vi "GetSwerveEncoders.vi"() -> (16 "Swerve 0 Velocity (ft/s)":dbl, 17 "Swerve 3 Velocity (ft/s)":dbl, 18 "Swerve 1 Velocity (ft/s)":dbl, 19 "Swerve 2 Velocity (ft/s)":dbl, 20 "Swerve 0 Azimuth Position (deg)":dbl, 22 "Swerve 1 Azimuth Position (deg)":dbl, 24 "Swerve 2 Azimuth Position (deg)":dbl, 26 "Swerve 3 Azimuth Position (deg)":dbl)   [LabVIEW 2020]
doc: "Gets the drive distance, azimuth position, and velocity encoder readings from all of the swerve modules. This VI is also useful for characterizing the drive system allowing for estimation of the robot acceleration and plotting of the module velocities. Deteremines the true shifter state based on photo-interrupter sensors on each module. Please see sensors.vi for a reading of the true robot ground speed (as this must be calculated after using the module odometry VIs)."
uses:
  driverdata.vi
  refnums.vi
  GRNF_CTREMotor.vi
  <vilib>/Rock Robotics/WPI/ThirdParty/Phoenix-LabVIEW/Motor Controller/Get/CTRE_Phoenix_MotorController_GetGeneralStatus.vi
  <vilib>/Rock Robotics/WPI/ThirdParty/Phoenix-LabVIEW/Motor Controller/Get/CTRE_Phoenix_MotorController_GetLimitSwitchStates.vi
  <vilib>/Rock Robotics/WPI/ThirdParty/Phoenix-LabVIEW/Motor Controller/Get/CTRE_Phoenix_MotorController_GetSelectedSensorData.vi
  sensors.vi
panel:
  in  "Shift Time Threshold (ms)":u32=250
  out "Acceleration (ft/s^2)":dbl format="%.1f"
  in  "Reset Acceleration Test":bool
  in  "Plot and Measure":bool
  out "Drive Encoder Velocities (ft/s)":cluster{dbl, dbl, dbl, dbl}(graph)
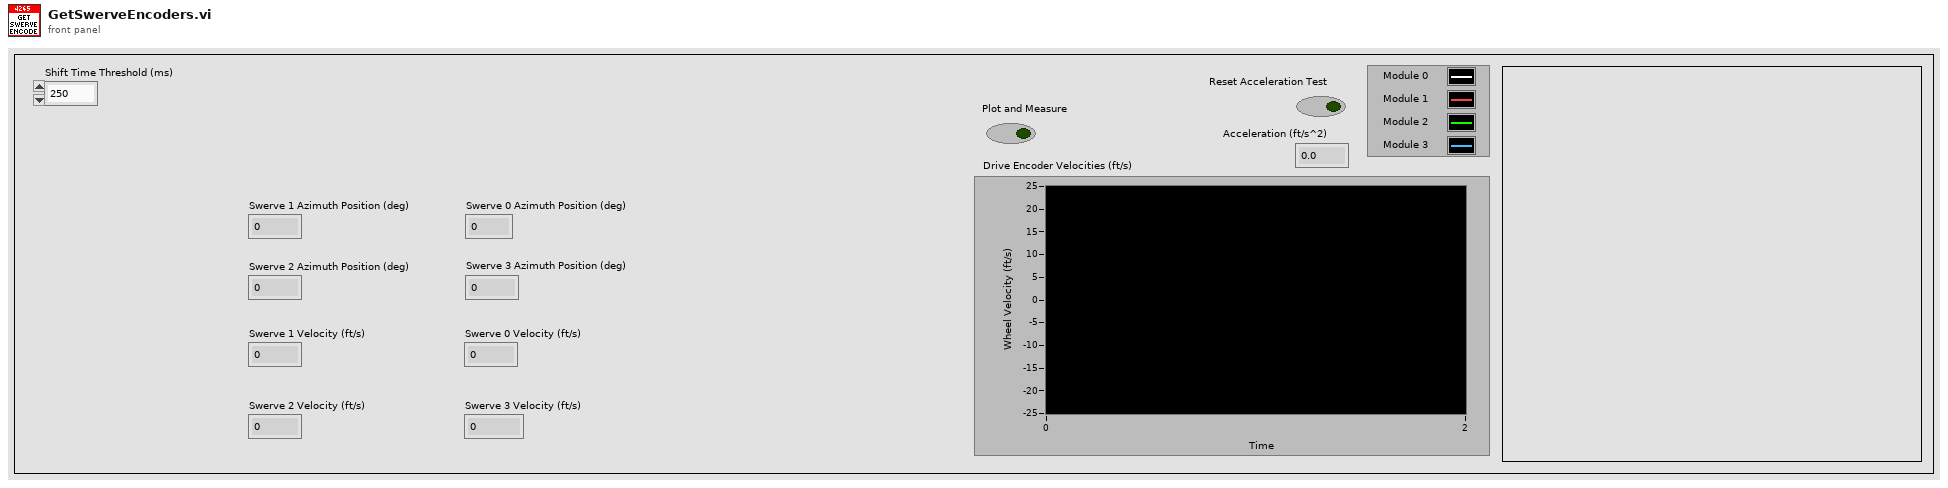
[diagram p1: front panel]
types:
  T1 = typedef "WPI_MotorControlDeviceRef.ctl" = cluster{"DeviceStatus":errorcluster, "Type":T2, "PWM":cluster{"PWM Channel":T3, "DeadBand":T4}, "CAN":cluster{"Device Number":u8, "SetOutput VI Ref":variant, "GetOutput VI Ref":variant, "Enable VI Ref":variant, "Disable VI Ref":variant, "Data":variant}, "Invert":bool, "DIO PWM":cluster{"PWM \"Enable\" Channel":T3, "DIOChannel":T5, "PWM Rate":dbl}}
  T2 = typedef "WPI_MotorControlType.ctl" = enum16{"PWM", "CAN", "DIO PWM"}
  T3 = typedef "FPGA_DIOPWMChannel.ctl" = enum8{"PWM 0", "PWM 1", "PWM 2", "PWM 3", "PWM 4", "PWM 5", "PWM 6", "PWM 7", "PWM 8", "PWM 9", "PWM MXP 0", "PWM MXP 1", "PWM MXP 2", "PWM MXP 3", "PWM MXP 4", "PWM MXP 5", "PWM MXP 6", "PWM MXP 7", "PWM MXP 8", "PWM MXP 9", "Invalid"}
  T4 = typedef "WPI_PWMDeadband.ctl" = cluster{"Name":string, "maxPositivePwm":i32, "minPositivePwm":i32, "centerPwm":i32, "maxNegativePwm":i32, "minNegativePwm":i32, "angularRange":u16}
  T5 = typedef "FPGA_DIOChannel.ctl" = enum8{"DIO 0", "DIO 1", "DIO 2", "DIO 3", "DIO 4", "DIO 5", "DIO 6", "DIO 7", "DIO 8", "DIO 9", "DIO MXP 0", "DIO MXP 1", "DIO MXP 2", "DIO MXP 3", "DIO MXP 4", "DIO MXP 5", "DIO MXP 6", "DIO MXP 7", "DIO MXP 8", "DIO MXP 9", "DIO MXP 10", "DIO MXP 11", "DIO MXP 12", "DIO MXP 13", "DIO MXP 14", "DIO MXP 15", "SPI Port CS1", "SPI Port CS2", "SPI Port CS3", "SPI Port MISO", "SPI Port MOSI", "Invalid"}
  T6 = enum16{"Low Gear", "High Gear", "Transiting", "Unknown", "Force Low Gear"}
  T7 = cluster{"Velocity (ft/s)":dbl, "Velocity (ft/s)":dbl, "Velocity (ft/s)":dbl, "Velocity (ft/s)":dbl}
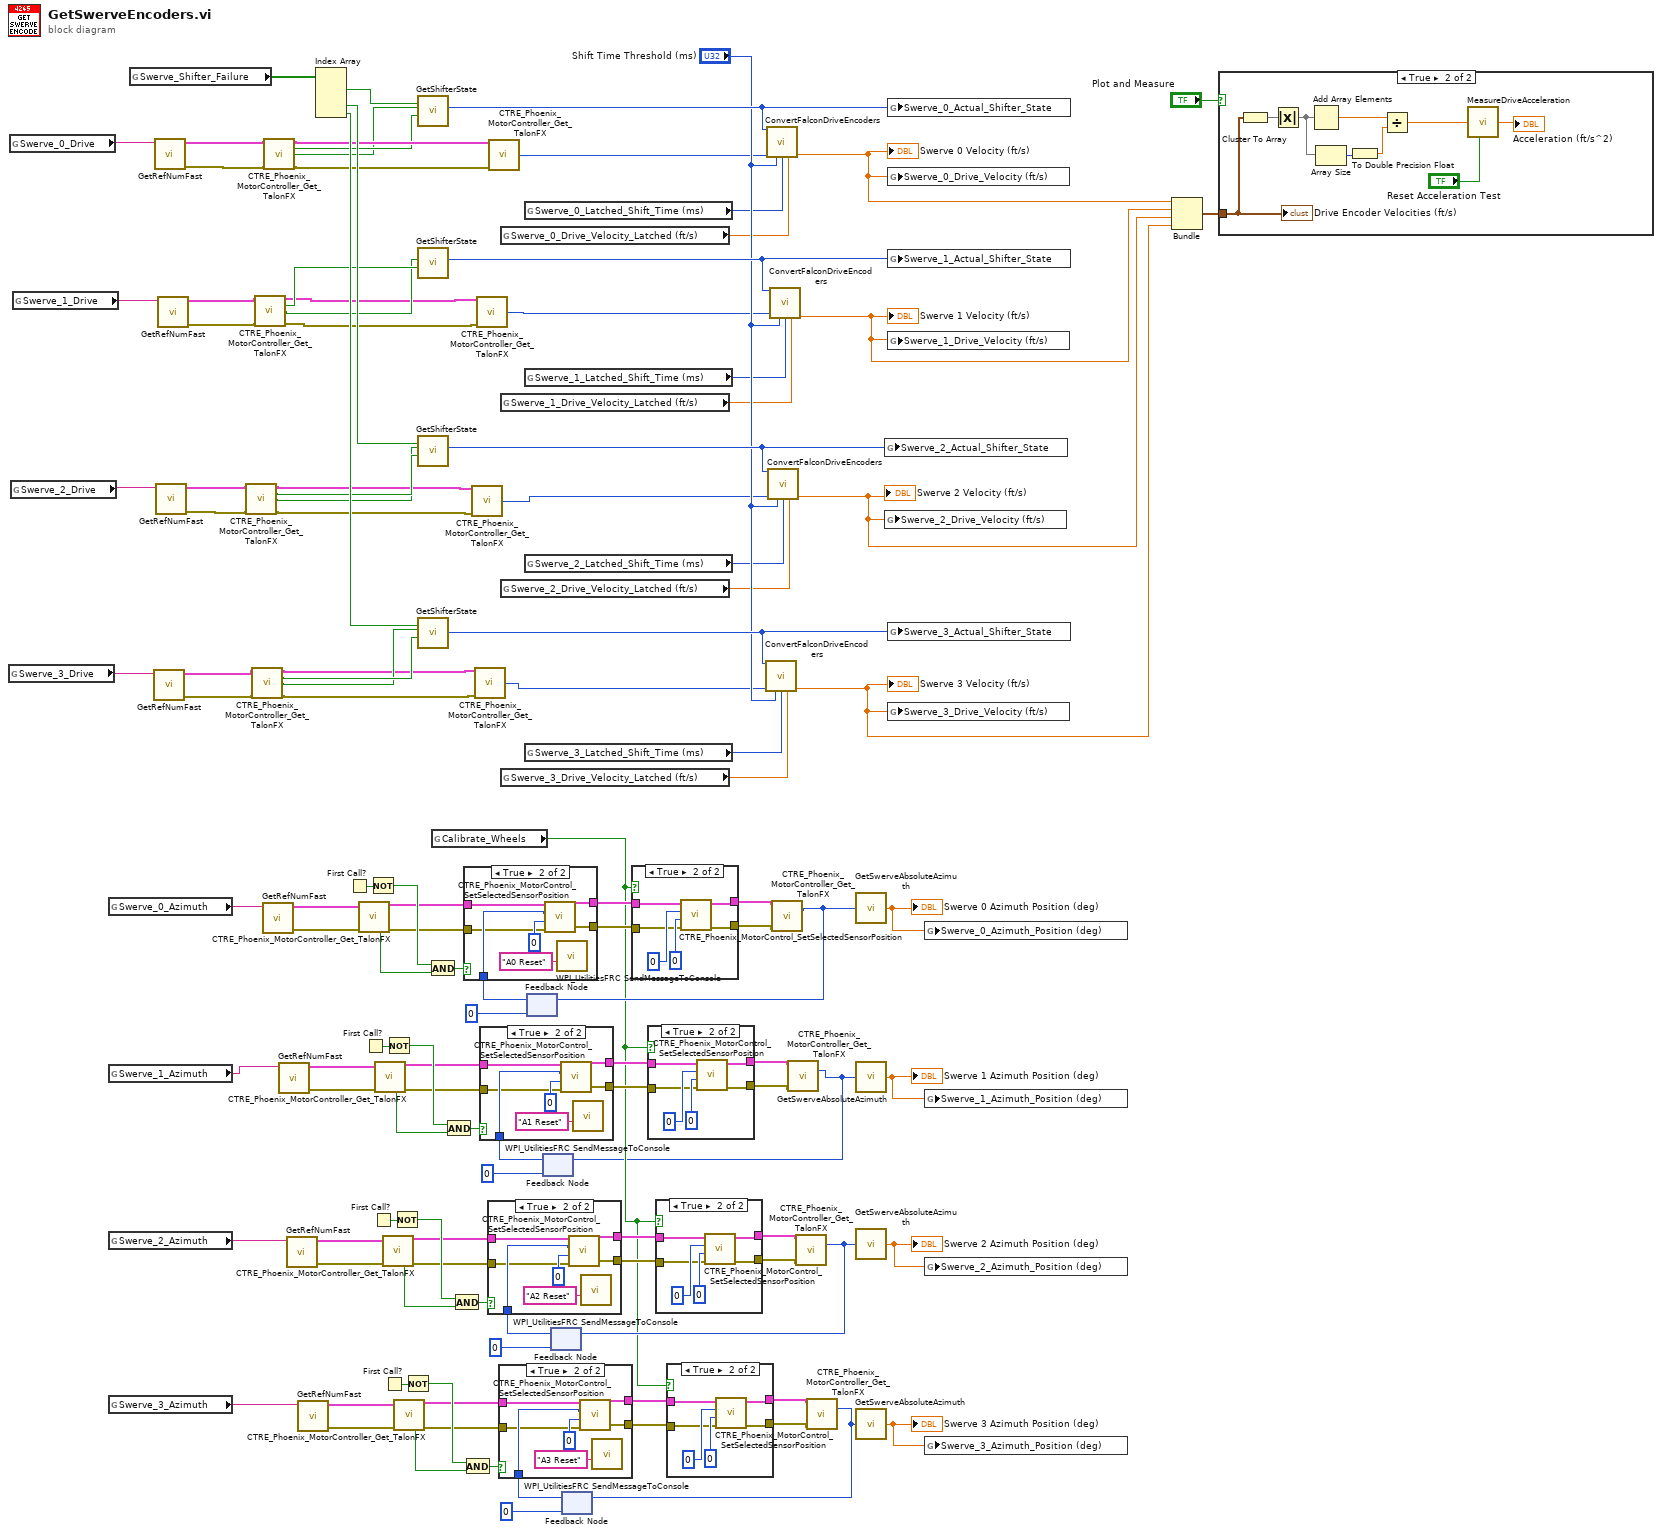
[diagram p0: block diagram]
diagram:
  n1 = global read "refnums.vi" "Swerve_3_Drive"() -> (w115:string)
  n2 = global read "refnums.vi" "Swerve_0_Drive"() -> (w118:string)
  n3 = global read "refnums.vi" "Swerve_2_Drive"() -> (w116:string)
  n4 = global read "refnums.vi" "Swerve_1_Drive"() -> (w117:string)
  n5 = global read "refnums.vi" "Swerve_0_Azimuth"() -> (w107:string)
  n6 = global read "refnums.vi" "Swerve_1_Azimuth"() -> (w63:string)
  n7 = global read "refnums.vi" "Swerve_2_Azimuth"() -> (w48:string)
  n8 = global read "refnums.vi" "Swerve_3_Azimuth"() -> (w32:string)
  n9 = global read "sensors.vi" "Swerve_Shifter_Failure"() -> (w114:bool[])
  n10 = call-poly "GetRefNumFast.vi"("RefNum Name"=w115) -> ("Error"=w4:errorcluster, "Device Reference"=w3:T1)  [unwired: 5 in]
  n11 = call-poly "GetRefNumFast.vi"("RefNum Name"=w118) -> ("Error"=w22:errorcluster, "Device Reference"=w21:T1)  [unwired: 5 in]
  n12 = call-poly "GetRefNumFast.vi"("RefNum Name"=w116) -> ("Error"=w10:errorcluster, "Device Reference"=w9:T1)  [unwired: 5 in]
  n13 = call-poly "GetRefNumFast.vi"("RefNum Name"=w117) -> ("Error"=w19:errorcluster, "Device Reference"=w20:T1)  [unwired: 5 in]
  n14 = call-poly <vilib>:"CTRE_Phoenix_MotorController_Get_TalonFX.vi"("PhoenixMotorControlDevRef"=w9, "error in"=w10) -> ("PhoenixMotorControlDevRef"=w12:T1, "Forward Limit Closed?"=w14:bool, "Reverse Limit Closed?"=w13:bool, "error out"=w11:errorcluster)  [unwired: 10 in]
  n15 = call-poly <vilib>:"CTRE_Phoenix_MotorController_Get_TalonFX.vi"("PhoenixMotorControlDevRef"=w3, "error in"=w4) -> ("PhoenixMotorControlDevRef"=w6:T1, "Forward Limit Closed?"=w8:bool, "Reverse Limit Closed?"=w7:bool, "error out"=w5:errorcluster)  [unwired: 10 in]
  n16 = call-poly <vilib>:"CTRE_Phoenix_MotorController_Get_TalonFX.vi"("PhoenixMotorControlDevRef"=w20, "error in"=w19) -> ("PhoenixMotorControlDevRef"=w16:T1, "Forward Limit Closed?"=w18:bool, "Reverse Limit Closed?"=w17:bool, "error out"=w15:errorcluster)  [unwired: 10 in]
  n17 = call-poly "GetRefNumFast.vi"("RefNum Name"=w107) -> ("Error"=w84:errorcluster, "Device Reference"=w85:T1)  [unwired: 5 in]
  n18 = call-poly <vilib>:"CTRE_Phoenix_MotorController_Get_TalonFX.vi"("PhoenixMotorControlDevRef"=w21, "error in"=w22) -> ("PhoenixMotorControlDevRef"=w25:T1, "Forward Limit Closed?"=w24:bool, "Reverse Limit Closed?"=w1:bool, "error out"=w23:errorcluster)  [unwired: 10 in]
  n19 = call-poly "GetRefNumFast.vi"("RefNum Name"=w63) -> ("Error"=w69:errorcluster, "Device Reference"=w70:T1)  [unwired: 5 in]
  n20 = call-poly "GetRefNumFast.vi"("RefNum Name"=w48) -> ("Error"=w54:errorcluster, "Device Reference"=w55:T1)  [unwired: 5 in]
  n21 = call-poly "GetRefNumFast.vi"("RefNum Name"=w32) -> ("Error"=w38:errorcluster, "Device Reference"=w39:T1)  [unwired: 5 in]
  n22 = Index Array(array=w114) -> (element #1=w113:bool, element #3=w112:bool, element #4=w111:bool)  [unwired: 4 in, 1 out]
  n23 = First Call?() -> (First Call?: T/F=w88:bool)
  n24 = call-poly <vilib>:"CTRE_Phoenix_MotorController_Get_TalonFX.vi"("PhoenixMotorControlDevRef"=w85, "error in"=w84) -> ("PhoenixMotorControlDevRef"=w83:T1, "Has Reset Occurred?"=w81:bool, "error out"=w82:errorcluster)  [unwired: 8 in, 3 out]
  n25 = First Call?() -> (First Call?: T/F=w73:bool)
  n26 = Not(x=w88) -> (.not. x?=w86:bool)
  n27 = First Call?() -> (First Call?: T/F=w58:bool)
  n28 = call-poly <vilib>:"CTRE_Phoenix_MotorController_Get_TalonFX.vi"("PhoenixMotorControlDevRef"=w70, "error in"=w69) -> ("PhoenixMotorControlDevRef"=w68:T1, "Has Reset Occurred?"=w66:bool, "error out"=w67:errorcluster)  [unwired: 8 in, 3 out]
  n29 = First Call?() -> (First Call?: T/F=w42:bool)
  n30 = call-poly <vilib>:"CTRE_Phoenix_MotorController_Get_TalonFX.vi"("PhoenixMotorControlDevRef"=w55, "error in"=w54) -> ("PhoenixMotorControlDevRef"=w53:T1, "Has Reset Occurred?"=w51:bool, "error out"=w52:errorcluster)  [unwired: 8 in, 3 out]
  n31 = Not(x=w73) -> (.not. x?=w71:bool)
  n32 = Not(x=w58) -> (.not. x?=w56:bool)
  n33 = call-poly <vilib>:"CTRE_Phoenix_MotorController_Get_TalonFX.vi"("PhoenixMotorControlDevRef"=w39, "error in"=w38) -> ("PhoenixMotorControlDevRef"=w37:T1, "Has Reset Occurred?"=w35:bool, "error out"=w36:errorcluster)  [unwired: 8 in, 3 out]
  n34 = Not(x=w42) -> (.not. x?=w40:bool)
  n35 = call "GetShifterState.vi"("Sensor Failure"=w113, "Low Gear Sensor"=w24, "High Gear Sensor"=w1) -> ("Actual Shifter State"=w104:T6)  [unwired: 8 in]
  n36 = call "GetShifterState.vi"("Low Gear Sensor"=w18, "High Gear Sensor"=w17) -> ("Actual Shifter State"=w105:T6)  [unwired: 9 in]
  n37 = call "GetShifterState.vi"("Sensor Failure"=w112, "Low Gear Sensor"=w14, "High Gear Sensor"=w13) -> ("Actual Shifter State"=w103:T6)  [unwired: 8 in]
  n38 = call "GetShifterState.vi"("Sensor Failure"=w111, "Low Gear Sensor"=w8, "High Gear Sensor"=w7) -> ("Actual Shifter State"=w102:T6)  [unwired: 8 in]
  n39 = And(x=w86, y=w81) -> (x .and. y?=w89:bool)
  n40 = global read "driverdata.vi" "Calibrate_Wheels"() -> (w31:bool)
  n41 = And(x=w71, y=w66) -> (x .and. y?=w74:bool)
  n42 = And(x=w56, y=w51) -> (x .and. y?=w59:bool)
  n43 = And(x=w40, y=w35) -> (x .and. y?=w43:bool)
  n44 = call-poly <vilib>:"CTRE_Phoenix_MotorController_Get_TalonFX.vi"("PhoenixMotorControlDevRef"=w12, "error in"=w11) -> ("Velocity (Raw Sensor Units per 100 ms)"=w27:i32)  [unwired: 10 in, 3 out]
  n45 = call-poly <vilib>:"CTRE_Phoenix_MotorController_Get_TalonFX.vi"("PhoenixMotorControlDevRef"=w6, "error in"=w5) -> ("Velocity (Raw Sensor Units per 100 ms)"=w26:i32)  [unwired: 10 in, 3 out]
  n46 = call-poly <vilib>:"CTRE_Phoenix_MotorController_Get_TalonFX.vi"("PhoenixMotorControlDevRef"=w16, "error in"=w15) -> ("Velocity (Raw Sensor Units per 100 ms)"=w28:i32)  [unwired: 10 in, 3 out]
  n47 = call-poly <vilib>:"CTRE_Phoenix_MotorController_Get_TalonFX.vi"("PhoenixMotorControlDevRef"=w25, "error in"=w23) -> ("Velocity (Raw Sensor Units per 100 ms)"=w29:i32)  [unwired: 10 in, 3 out]
  n48 = global read "sensors.vi" "Swerve_0_Drive_Velocity_Latched (ft/s)"() -> (w99:dbl)
  n49 = global read "sensors.vi" "Swerve_1_Drive_Velocity_Latched (ft/s)"() -> (w97:dbl)
  n50 = global read "sensors.vi" "Swerve_2_Drive_Velocity_Latched (ft/s)"() -> (w95:dbl)
  n51 = global read "sensors.vi" "Swerve_3_Drive_Velocity_Latched (ft/s)"() -> (w93:dbl)
  n52 = global read "sensors.vi" "Swerve_0_Latched_Shift_Time (ms)"() -> (w100:u32)
  n53 = global read "sensors.vi" "Swerve_1_Latched_Shift_Time (ms)"() -> (w98:u32)
  n54 = global read "sensors.vi" "Swerve_2_Latched_Shift_Time (ms)"() -> (w96:u32)
  n55 = global read "sensors.vi" "Swerve_3_Latched_Shift_Time (ms)"() -> (w94:u32)
  n56 = feedback #1(0 ("Position (Raw Sensor Units)")) -> (w92:i32)
  n57 = case shown="True" w89 {
    tunnel: w82 -> [w125 w129]
    tunnel: w83 -> [w126 w132]
    tunnel: [w126 w128] -> w91
    tunnel: [w125 w127] -> w90
    tunnel: w92 -> [_ w131]
    frame False {
    }
    frame True {
      n58 = call <vilib>:"CTRE_Phoenix_MotorControl_SetSelectedSensorPosition.vi"("error in (no error)"=w129, "pidLoopIdx"=u32 0, "New Sensor Position"=w131, "PhoenixMotorControlDevRef"=w132) -> ("error out"=w127:errorcluster, "PhoenixMotorControlDevRef"=w128:T1)  [unwired: 6 in]
      n59 = call <vilib>:"WPI_UtilitiesFRC SendMessageToConsole.vi"("Message"="A0 Reset") -> ()  [unwired: 14 in, 1 out]
    }
  }
  n60 = feedback #2(0 ("Position (Raw Sensor Units)")) -> (w77:i32)
  n61 = case shown="True" w74 {
    tunnel: w67 -> [w134 w138]
    tunnel: w68 -> [w135 w141]
    tunnel: [w135 w137] -> w76
    tunnel: [w134 w136] -> w75
    tunnel: w77 -> [_ w140]
    frame False {
    }
    frame True {
      n62 = call <vilib>:"CTRE_Phoenix_MotorControl_SetSelectedSensorPosition.vi"("error in (no error)"=w138, "pidLoopIdx"=u32 0, "New Sensor Position"=w140, "PhoenixMotorControlDevRef"=w141) -> ("error out"=w136:errorcluster, "PhoenixMotorControlDevRef"=w137:T1)  [unwired: 6 in]
      n63 = call <vilib>:"WPI_UtilitiesFRC SendMessageToConsole.vi"("Message"="A1 Reset") -> ()  [unwired: 14 in, 1 out]
    }
  }
  n64 = feedback #3(0 ("Position (Raw Sensor Units)")) -> (w62:i32)
  n65 = case shown="True" w59 {
    tunnel: w52 -> [w143 w147]
    tunnel: w53 -> [w144 w150]
    tunnel: [w144 w146] -> w61
    tunnel: [w143 w145] -> w60
    tunnel: w62 -> [_ w149]
    frame False {
    }
    frame True {
      n66 = call <vilib>:"CTRE_Phoenix_MotorControl_SetSelectedSensorPosition.vi"("error in (no error)"=w147, "pidLoopIdx"=u32 0, "New Sensor Position"=w149, "PhoenixMotorControlDevRef"=w150) -> ("error out"=w145:errorcluster, "PhoenixMotorControlDevRef"=w146:T1)  [unwired: 6 in]
      n67 = call <vilib>:"WPI_UtilitiesFRC SendMessageToConsole.vi"("Message"="A2 Reset") -> ()  [unwired: 14 in, 1 out]
    }
  }
  n68 = feedback #4(0 ("Position (Raw Sensor Units)")) -> (w46:i32)
  n69 = case shown="True" w43 {
    tunnel: w36 -> [w152 w156]
    tunnel: w37 -> [w153 w159]
    tunnel: [w153 w155] -> w45
    tunnel: [w152 w154] -> w44
    tunnel: w46 -> [_ w158]
    frame False {
    }
    frame True {
      n70 = call <vilib>:"CTRE_Phoenix_MotorControl_SetSelectedSensorPosition.vi"("error in (no error)"=w156, "pidLoopIdx"=u32 0, "New Sensor Position"=w158, "PhoenixMotorControlDevRef"=w159) -> ("error out"=w154:errorcluster, "PhoenixMotorControlDevRef"=w155:T1)  [unwired: 6 in]
      n71 = call <vilib>:"WPI_UtilitiesFRC SendMessageToConsole.vi"("Message"="A3 Reset") -> ()  [unwired: 14 in, 1 out]
    }
  }
  n72 = case shown="True" w31 {
    tunnel: w90 -> [w161 w163]
    tunnel: w91 -> [w162 w166]
    tunnel: [w162 w167] -> w80
    tunnel: [w161 w168] -> w79
    frame False {
    }
    frame True {
      n73 = call <vilib>:"CTRE_Phoenix_MotorControl_SetSelectedSensorPosition.vi"("error in (no error)"=w163, "pidLoopIdx"=u32 0, "New Sensor Position"=0, "PhoenixMotorControlDevRef"=w166) -> ("error out"=w168:errorcluster, "PhoenixMotorControlDevRef"=w167:T1)  [unwired: 6 in]
    }
  }
  n74 = case shown="True" w31 {
    tunnel: w75 -> [w169 w171]
    tunnel: w76 -> [w170 w174]
    tunnel: [w170 w175] -> w65
    tunnel: [w169 w176] -> w64
    frame False {
    }
    frame True {
      n75 = call <vilib>:"CTRE_Phoenix_MotorControl_SetSelectedSensorPosition.vi"("error in (no error)"=w171, "pidLoopIdx"=u32 0, "New Sensor Position"=0, "PhoenixMotorControlDevRef"=w174) -> ("error out"=w176:errorcluster, "PhoenixMotorControlDevRef"=w175:T1)  [unwired: 6 in]
    }
  }
  n76 = case shown="True" w31 {
    tunnel: w60 -> [w177 w179]
    tunnel: w61 -> [w178 w182]
    tunnel: [w178 w183] -> w50
    tunnel: [w177 w184] -> w49
    frame False {
    }
    frame True {
      n77 = call <vilib>:"CTRE_Phoenix_MotorControl_SetSelectedSensorPosition.vi"("error in (no error)"=w179, "pidLoopIdx"=u32 0, "New Sensor Position"=0, "PhoenixMotorControlDevRef"=w182) -> ("error out"=w184:errorcluster, "PhoenixMotorControlDevRef"=w183:T1)  [unwired: 6 in]
    }
  }
  n78 = case shown="True" w31 {
    tunnel: w44 -> [w185 w187]
    tunnel: w45 -> [w186 w190]
    tunnel: [w186 w191] -> w34
    tunnel: [w185 w192] -> w33
    frame False {
    }
    frame True {
      n79 = call <vilib>:"CTRE_Phoenix_MotorControl_SetSelectedSensorPosition.vi"("error in (no error)"=w187, "pidLoopIdx"=u32 0, "New Sensor Position"=0, "PhoenixMotorControlDevRef"=w190) -> ("error out"=w192:errorcluster, "PhoenixMotorControlDevRef"=w191:T1)  [unwired: 6 in]
    }
  }
  n80 = call "ConvertFalconDriveEncoders.vi"("Shifter State"=w102, "Velocity (Raw Sensor Units per 100 ms)"=w26, "Shift Time Threshold (ms)"="Shift Time Threshold (ms)", "Latched Shift Time (ms)"=w94, "Latched Velocity (ft/s)"=w93) -> ("Velocity (ft/s)"=w119:dbl)  [unwired: 10 in]
  "Swerve 3 Velocity (ft/s)" <- w119
  n81 = call "ConvertFalconDriveEncoders.vi"("Shifter State"=w104, "Velocity (Raw Sensor Units per 100 ms)"=w29, "Shift Time Threshold (ms)"="Shift Time Threshold (ms)", "Latched Shift Time (ms)"=w100, "Latched Velocity (ft/s)"=w99) -> ("Velocity (ft/s)"=w123:dbl)  [unwired: 10 in]
  "Swerve 0 Velocity (ft/s)" <- w123
  n82 = call "ConvertFalconDriveEncoders.vi"("Shifter State"=w103, "Velocity (Raw Sensor Units per 100 ms)"=w27, "Shift Time Threshold (ms)"="Shift Time Threshold (ms)", "Latched Shift Time (ms)"=w96, "Latched Velocity (ft/s)"=w95) -> ("Velocity (ft/s)"=w120:dbl)  [unwired: 10 in]
  "Swerve 2 Velocity (ft/s)" <- w120
  n83 = call "ConvertFalconDriveEncoders.vi"("Shifter State"=w105, "Velocity (Raw Sensor Units per 100 ms)"=w28, "Shift Time Threshold (ms)"="Shift Time Threshold (ms)", "Latched Shift Time (ms)"=w98, "Latched Velocity (ft/s)"=w97) -> ("Velocity (ft/s)"=w121:dbl)  [unwired: 10 in]
  "Swerve 1 Velocity (ft/s)" <- w121
  n84 = call-poly <vilib>:"CTRE_Phoenix_MotorController_Get_TalonFX.vi"("PhoenixMotorControlDevRef"=w80, "error in"=w79) -> ("Position (Raw Sensor Units)"=w78:i32)  [unwired: 10 in, 3 out]
  n85 = feedback-in #1(w78) -> ()
  n86 = call-poly <vilib>:"CTRE_Phoenix_MotorController_Get_TalonFX.vi"("PhoenixMotorControlDevRef"=w65, "error in"=w64) -> ("Position (Raw Sensor Units)"=w2:i32)  [unwired: 10 in, 3 out]
  n87 = feedback-in #2(w2) -> ()
  n88 = call-poly <vilib>:"CTRE_Phoenix_MotorController_Get_TalonFX.vi"("PhoenixMotorControlDevRef"=w50, "error in"=w49) -> ("Position (Raw Sensor Units)"=w47:i32)  [unwired: 10 in, 3 out]
  n89 = feedback-in #3(w47) -> ()
  n90 = call-poly <vilib>:"CTRE_Phoenix_MotorController_Get_TalonFX.vi"("PhoenixMotorControlDevRef"=w34, "error in"=w33) -> ("Position (Raw Sensor Units)"=w30:i32)  [unwired: 10 in, 3 out]
  n91 = feedback-in #4(w30) -> ()
  n92 = call "GetSwerveAbsoluteAzimuth.vi"("Relative Position (Raw Sensor Units)"=w78) -> ("Azimuth Position (deg) [-180,+180]"=w106:dbl)
  "Swerve 0 Azimuth Position (deg)" <- w106
  n93 = call "GetSwerveAbsoluteAzimuth.vi"("Relative Position (Raw Sensor Units)"=w2) -> ("Azimuth Position (deg) [-180,+180]"=w108:dbl)
  "Swerve 1 Azimuth Position (deg)" <- w108
  n94 = call "GetSwerveAbsoluteAzimuth.vi"("Relative Position (Raw Sensor Units)"=w47) -> ("Azimuth Position (deg) [-180,+180]"=w109:dbl)
  "Swerve 2 Azimuth Position (deg)" <- w109
  n95 = call "GetSwerveAbsoluteAzimuth.vi"("Relative Position (Raw Sensor Units)"=w30) -> ("Azimuth Position (deg) [-180,+180]"=w110:dbl)
  "Swerve 3 Azimuth Position (deg)" <- w110
  n96 = global write "sensors.vi" "Swerve_2_Actual_Shifter_State"(w103) -> ()
  n97 = global write "sensors.vi" "Swerve_2_Drive_Velocity (ft/s)"(w120) -> ()
  n98 = global write "sensors.vi" "Swerve_0_Actual_Shifter_State"(w104) -> ()
  n99 = global write "sensors.vi" "Swerve_0_Drive_Velocity (ft/s)"(w123) -> ()
  n100 = global write "sensors.vi" "Swerve_1_Actual_Shifter_State"(w105) -> ()
  n101 = global write "sensors.vi" "Swerve_1_Drive_Velocity (ft/s)"(w121) -> ()
  n102 = global write "sensors.vi" "Swerve_3_Actual_Shifter_State"(w102) -> ()
  n103 = global write "sensors.vi" "Swerve_3_Drive_Velocity (ft/s)"(w119) -> ()
  n104 = global write "sensors.vi" "Swerve_0_Azimuth_Position (deg)"(w106) -> ()
  n105 = global write "sensors.vi" "Swerve_1_Azimuth_Position (deg)"(w108) -> ()
  n106 = global write "sensors.vi" "Swerve_2_Azimuth_Position (deg)"(w109) -> ()
  n107 = global write "sensors.vi" "Swerve_3_Azimuth_Position (deg)"(w110) -> ()
  n108 = Bundle("Velocity (ft/s)"=w123, "Velocity (ft/s)"=w121, "Velocity (ft/s)"=w120, "Velocity (ft/s)"=w119) -> (w122:T7)  [unwired: 1 in]
  n109 = case shown="True" "Plot and Measure" {
    tunnel: w122 -> [_ w196]
    frame False {
    }
    frame True {
      n110 = Cluster To Array(cluster=w196) -> (array=w198:dbl[])
      n111 = Absolute Value(x=w198) -> (abs(x)=w201:dbl[])
      n112 = Add Array Elements(numeric array=w201) -> (sum=w197:dbl)
      n113 = Array Size(array=w201) -> (size(s)=w199:i32)
      n114 = To Double Precision Float(number=w199) -> (double precision float=w200:dbl)
      n115 = Divide(x=w197, y=w200) -> (x/y=w195:dbl)
      n116 = call "MeasureDriveAcceleration.vi"("Average Drive Velocity (ft/s)"=w195, "Reset"="Reset Acceleration Test") -> ("Acceleration (ft/s^2)"=→"Acceleration (ft/s^2)":dbl)  [unwired: 3 in]
      "Drive Encoder Velocities (ft/s)" <- w196
    }
  }
